vi "search for ID.vi"(10 "instance id":string, 11 "instance data":refnum<class "NISE_CEF_serializable configuration.lvclass">[](array[class])) -> (3 "index":i32)   [LabVIEW 2013, in "NISE_CEF_serializable configuration.lvclass"]
uses:
  serializable configuration/NISE_CEF_serializable configuration.lvclass
  serializable configuration/NISE_CEF_serializable configuration.lvclass/NISE_CEF_serializable configuration.ctl
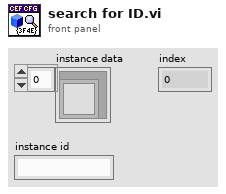
[diagram p1: front panel]
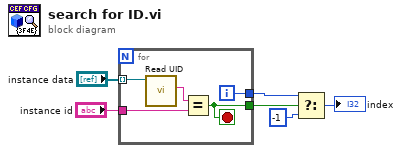
[diagram p0: block diagram]
diagram:
  n1 = for {
    tunnel: "instance data" -> [w7] mode=indexing
    tunnel: "instance id" -> [w10]
    tunnel: [w9] -> w2
    tunnel: [w8] -> w4
    i -> [w9]
    stop <- w8 stop-if-true
    n2 = call "Read UID.vi"("configuration in"=w7) -> ("instance id"=w11:string)  [unwired: 8 in, 2 out]
    n3 = Equal?(x=w11, y=w10) -> (x = y?=w8:bool)
  }
  n4 = Select(t=w2, s=w4, f=-1) -> (s? t:f=→"index":i32)
